vi "test_pearson_map.vi"() -> ()   [LabVIEW 2009]
doc: "Copyright (C) 2009, Stepan A. Baranov\nweb: http://www.OCTLab.org/\nemail: stepan@baranov.su"
uses:
  <vilib>/gmath/NI_Gmath.lvlib
  OCTLib.dll
panel:
  out "vertical radius":i32
  out "error out":errorcluster
  out "horizontal radius":i32
  out "width":i32
  out "height":i32
  in  "Small/Big":bool
  out "loop #":i32
  out "RSM_STAT time":u32
  out "LabView time":u32
  out "RSM_STAT Array":dbl[][](array[numeric])
  out "LabView Array":dbl[][](array[numeric])
  in  "stop":bool
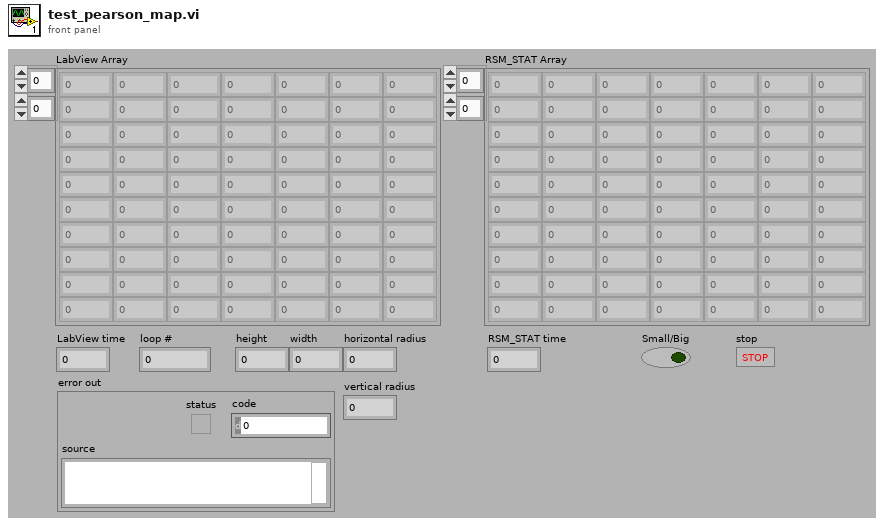
[diagram p1: front panel]
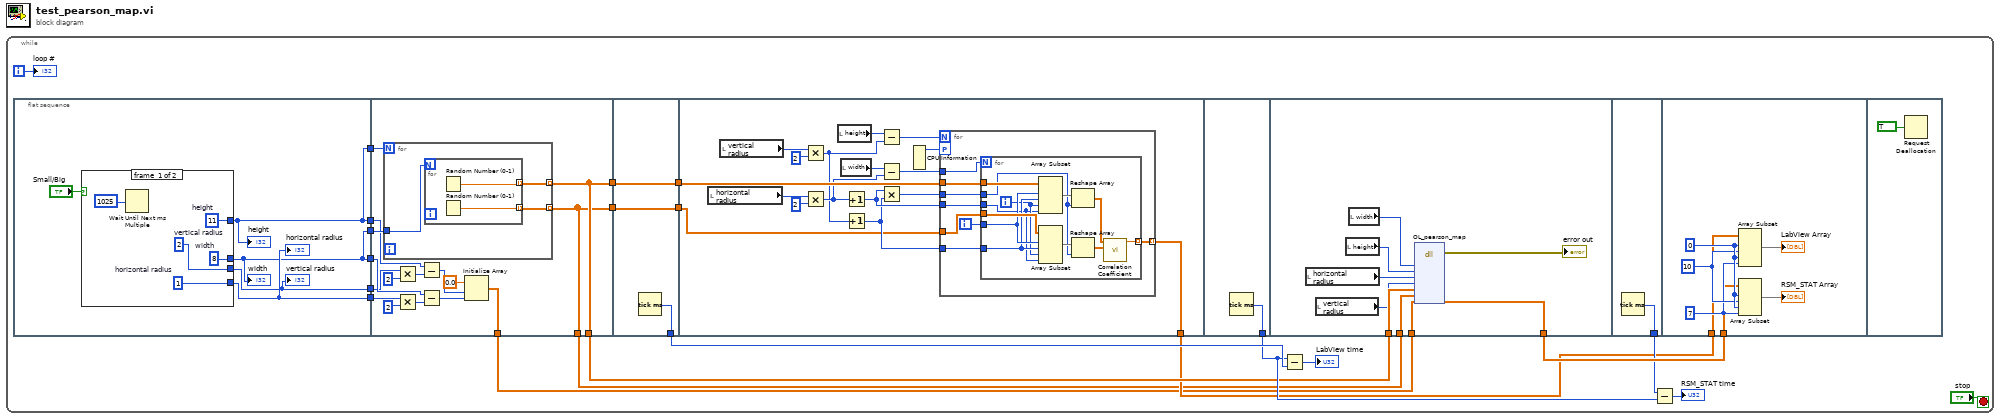
[diagram p0: block diagram]
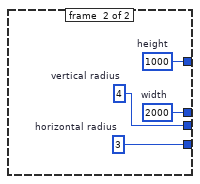
[diagram p2: hidden frame]
diagram:
  n1 = while {
    i -> [w15]
    stop <- "stop" stop-if-true
    n2 = flat-sequence {
      tunnel: [w24] -> w11
      tunnel: [w25] -> w10
      tunnel: [w26] -> w8
      tunnel: [w25] -> w7
      tunnel: [w24] -> w6
      tunnel: [w23] -> w4
      tunnel: [w50] -> w14
      tunnel: [w50] -> w12
      tunnel: w11 -> [w52]
      tunnel: w10 -> [w51]
      tunnel: w8 -> [w48]
      tunnel: w7 -> [w46]
      tunnel: w6 -> [w44]
      tunnel: [w41] -> w5
      tunnel: w4 -> [w39]
      tunnel: [w37] -> w3
      tunnel: [w37] -> w1
      tunnel: [w60] -> w20
      tunnel: [w59] -> w13
      tunnel: w12 -> [w59]
      tunnel: w3 -> [w58]
      tunnel: [w58] -> w2
      tunnel: w13 -> [w77]
      tunnel: [w73] -> w9
      tunnel: w2 -> [w61]
      tunnel: [w98] -> w17
      tunnel: w14 -> [w106]
      tunnel: [w105] -> w21
      tunnel: w5 -> [w107]
      tunnel: w1 -> [w99]
      tunnel: [w108] -> w18
      tunnel: w21 -> [w111]
      tunnel: w9 -> [w110]
      frame #0 {
        n3 = case shown="False" "Small/Big" {
          tunnel: [w30 w36] -> w25
          tunnel: [w31 w35] -> w24
          tunnel: [w32 w34] -> w26
          tunnel: [w28 w33] -> w23
          frame #0 {
            w28 = 2  # vertical radius
            w32 = 1  # horizontal radius
            w31 = 8  # width
            w30 = 11  # height
            n4 = Wait Until Next ms Multiple(millisecond multiple=u32 1025) -> ()  [unwired: 1 out]
          }
          frame #1 {
            w33 = 4  # vertical radius
            w34 = 3  # horizontal radius
            w35 = 2000  # width
            w36 = 1000  # height
          }
        }
        "height" <- w25
        "width" <- w24
        "horizontal radius" <- w26
        "vertical radius" <- w23
      }
      frame #1 {
        n5 = for {
          N: w51 -> [_]
          tunnel: w52 -> [w55]
          tunnel: [w54] -> w50 mode=indexing
          tunnel: [w53] -> w37 mode=indexing
          n6 = for {
            N: w55 -> [_]
            tunnel: [w57] -> w54 mode=indexing
            tunnel: [w56] -> w53 mode=indexing
            n7 = Random Number (0-1)() -> (number: 0 to 1=w57:dbl)
            n8 = Random Number (0-1)() -> (number: 0 to 1=w56:dbl)
          }
        }
        n9 = Multiply(x=w39, y=2) -> (x*y=w38:i32)
        n10 = Multiply(x=w48, y=2) -> (x*y=w43:i32)
        n11 = Subtract(x=w46, y=w38) -> (x-y=w45:i32)
        n12 = Subtract(x=w44, y=w43) -> (x-y=w42:i32)
        n13 = Initialize Array(0.0 ("element"), w45, w42) -> (w41:dbl[][])
      }
      frame #2 {
        n14 = Tick Count (ms)() -> (millisecond timer value=w60:u32)
      }
      frame #3 {
        n15 = local read "horizontal radius"() -> (w76:i32)
        n16 = local read "vertical radius"() -> (w65:i32)
        n17 = Multiply(x=w65, y=2) -> (x*y=w63:i32)
        n18 = Multiply(x=w76, y=2) -> (x*y=w69:i32)
        n19 = local read "height"() -> (w72:i32)
        n20 = local read "width"() -> (w70:i32)
        n21 = Increment(x=w69) -> (x+1=w64:i32)
        n22 = Increment(x=w63) -> (x+1=w62:i32)
        n23 = Subtract(x=w72, y=w63) -> (x-y=w71:i32)
        n24 = Subtract(x=w70, y=w69) -> (x-y=w68:i32)
        n25 = Multiply(x=w64, y=w62) -> (x*y=w74:i32)
        n26 = CPU Information() -> (4:w67:i32)  [unwired: 3 out]
        n27 = for {
          N: w71 -> [_]
          tunnel: w77 -> [w84]
          tunnel: w74 -> [w83]
          tunnel: [w82] -> w73 mode=indexing
          tunnel: w64 -> [w81]
          tunnel: w68 -> [w80]
          workers-P: w67 -> [_]
          tunnel: w62 -> [w79]
          tunnel: w61 -> [w78]
          i -> [w85]
          n28 = for {
            N: w80 -> [_]
            tunnel: w85 -> [w93]
            tunnel: w84 -> [w97]
            tunnel: w83 -> [w89]
            tunnel: [w86] -> w82 mode=indexing
            tunnel: w81 -> [w90]
            tunnel: w79 -> [w92]
            tunnel: w78 -> [w94]
            i -> [w91]
            n29 = Array Subset(array=w97, index (row)=w93, length (row)=w92, index (col)=w91, length (col)=w90) -> (w96:dbl[][])
            n30 = Array Subset(array=w94, index (row)=w93, length (row)=w92, index (col)=w91, length (col)=w90) -> (w95:dbl[][])
            n31 = Reshape Array(w96, w89) -> (w88:dbl[])
            n32 = Reshape Array(w95, w89) -> (w87:dbl[])
            n33 = call <vilib>:"Correlation Coefficient.vi"("Y"=w87, "X"=w88) -> ("correlation coefficient r"=w86:dbl)  [unwired: 8 in, 1 out]
          }
        }
      }
      frame #4 {
        n34 = Tick Count (ms)() -> (millisecond timer value=w98:u32)
      }
      frame #5 {
        n35 = local read "horizontal radius"() -> (w101:i32)
        n36 = local read "vertical radius"() -> (w100:i32)
        n37 = local read "height"() -> (w103:i32)
        n38 = local read "width"() -> (w104:i32)
        n39 = dll-call lib="OCTLib.dll" fn="OL_pearson_map"("width"=w104, "height"=w103, "horizontal radius"=w101, "vertical radius"=w100, "input1"=w106, "input2"=w99, "output"=w107) -> (error out=→"error out":errorcluster, "output"=w105:dbl[][])  [unwired: 10 in, 1 out]
      }
      frame #6 {
        n40 = Tick Count (ms)() -> (millisecond timer value=w108:u32)
      }
      frame #7 {
        w114 = 10 ("length")
        w113 = 7 ("length")
        w115 = 0 ("index")
        n41 = Array Subset(array=w110, index (row)=w115, length (row)=w114, index (col)=w115, length (col)=w113) -> (→"LabView Array":dbl[][])
        n42 = Array Subset(array=w111, index (row)=w115, length (row)=w114, index (col)=w115, length (col)=w113) -> (→"RSM_STAT Array":dbl[][])
      }
      frame #8 {
        n43 = Request Deallocation(TRUE ("flag")) -> ()
      }
    }
    n44 = Subtract(x=w17, y=w20) -> (x-y=→"LabView time":u32)
    n45 = Subtract(x=w18, y=w17) -> (x-y=→"RSM_STAT time":u32)
    "loop #" <- w15
  }
